vi "BuildPlotLegends_LSI218.vi"(8 "Plot selecter (2)\n    1      2     3     5":bool[][](array[boolean])=[[FALSE, TRUE, FALSE, FALSE], [FALSE, FALSE, FALSE, FALSE], [FALSE, FALSE, FALSE, FALSE], [FALSE, FALSE, FALSE, TRUE], [TRUE, FALSE, FALSE, FALSE], [FALSE, FALSE, FALSE, FALSE], [FALSE, FALSE, FALSE, FALSE], [FALSE, TRUE, FALSE, FALSE], [FALSE, TRUE, FALSE, FALSE], [FALSE, TRUE, FALSE, FALSE], [FALSE, TRUE, FALSE, FALSE], [FALSE, FALSE, FALSE, FALSE], [FALSE, FALSE, FALSE, FALSE], [FALSE, FALSE, FALSE, FALSE], [FALSE, FALSE, FALSE, FALSE], [FALSE, FALSE, FALSE, FALSE], [FALSE, FALSE, FALSE, FALSE], [FALSE, FALSE, FALSE, FALSE], [FALSE, FALSE, FALSE, FALSE], [FALSE, FALSE, FALSE, FALSE], [FALSE, FALSE, FALSE, FALSE], [FALSE, FALSE, FALSE, FALSE], [FALSE, FALSE, FALSE, FALSE], [FALSE, FALSE, FALSE, FALSE]], 9 "Plot selecter (1)\n    1      2     3     4":bool[][](array[boolean])=[[FALSE, TRUE, FALSE, FALSE], [FALSE, FALSE, FALSE, FALSE], [FALSE, FALSE, FALSE, FALSE], [FALSE, FALSE, FALSE, TRUE], [TRUE, FALSE, FALSE, FALSE], [FALSE, FALSE, FALSE, FALSE], [FALSE, FALSE, FALSE, FALSE], [FALSE, TRUE, FALSE, FALSE], [FALSE, TRUE, FALSE, FALSE], [FALSE, TRUE, FALSE, FALSE], [FALSE, TRUE, FALSE, FALSE], [FALSE, FALSE, FALSE, FALSE], [FALSE, FALSE, FALSE, FALSE], [FALSE, FALSE, FALSE, FALSE], [FALSE, FALSE, FALSE, FALSE], [FALSE, FALSE, FALSE, FALSE], [FALSE, FALSE, FALSE, FALSE], [FALSE, FALSE, FALSE, FALSE], [FALSE, FALSE, FALSE, FALSE], [FALSE, FALSE, FALSE, FALSE], [FALSE, FALSE, FALSE, FALSE], [FALSE, FALSE, FALSE, FALSE], [FALSE, FALSE, FALSE, FALSE], [FALSE, FALSE, FALSE, FALSE]], 10 "Labels (2)":string[](array[string])=["B1", "B2", "B3", "B4", "B5"], 11 "Labels (1)":string[](array[string])=["A1", "A2", "A3", "A4", "A5"]) -> (0 "Series 4":string[](array[string])=["A4"], 1 "Series 3":string[](array[string]), 2 "Series 2":string[](array[string])=["A1", "B3", "B4", "B5"], 3 "Series 1":string[](array[string])=["A5"])   [LabVIEW 2017]
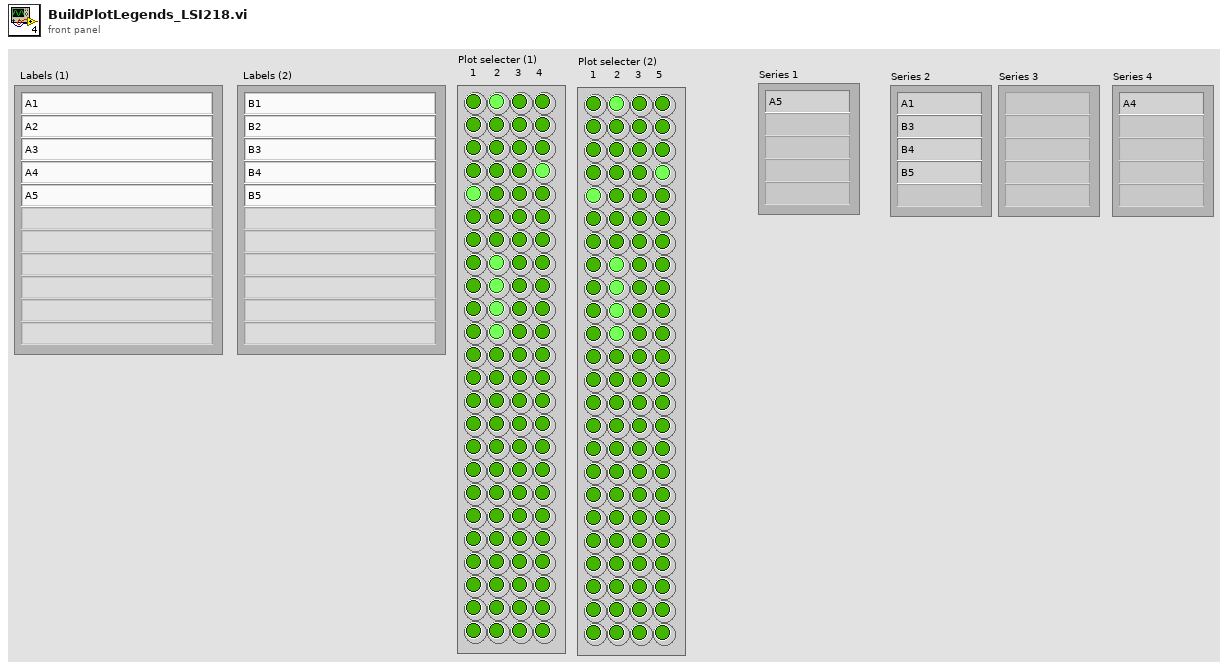
[diagram p1: front panel]
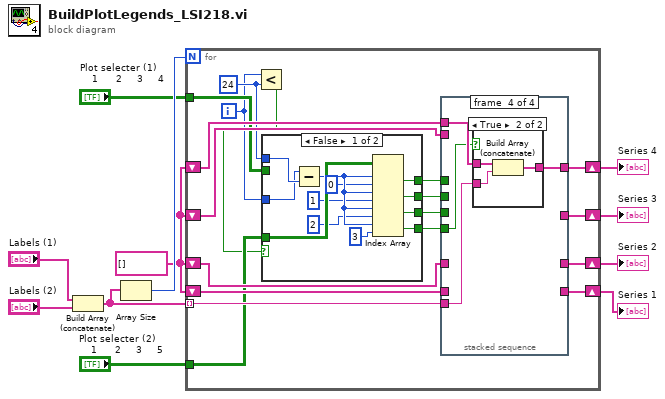
[diagram p0: block diagram]
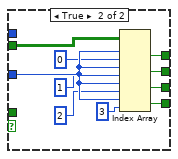
[diagram p2: hidden frame]
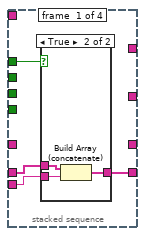
[diagram p3: hidden frame]
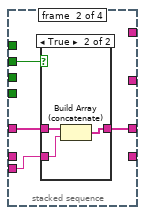
[diagram p5: hidden frame]
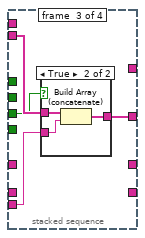
[diagram p7: hidden frame]
diagram:
  w9 = string[] []
  n1 = Build Array (concatenate)("Labels (1)", "Labels (2)") -> (w2:string[])
  n2 = Array Size(array=w2) -> (size(s)=w11:i32)
  n3 = for {
    N: w11 -> [_]
    shift-right: [w22] -> w8
    shift-left: w9 -> [w29]
    shift-right: [w24] -> w6
    shift-left: w9 -> [w28]
    shift-right: [w23] -> w7
    shift-left: w9 -> [w27]
    shift-right: [w21] -> w5
    shift-left: w9 -> [w26]
    tunnel: "Plot selecter (1)\n    1      2     3     4" -> [w19]
    tunnel: w2 -> [w25] mode=indexing
    tunnel: "Plot selecter (2)\n    1      2     3     5" -> [w18]
    i -> [w13]
    w20 = 24 ("y")
    n4 = Less?(x=w13, y=w20) -> (x < y?=w12:bool)
    n5 = case shown="False" w12 {
      tunnel: [w33 w51] -> w17
      tunnel: [w32 w50] -> w16
      tunnel: [w31 w48] -> w15
      tunnel: [w30 w47] -> w14
      tunnel: w20 -> [w40 _]
      tunnel: w19 -> [_ w46]
      tunnel: w18 -> [w39 _]
      tunnel: w13 -> [w34 w45]
      frame False {
        n6 = Subtract(x=w34, y=w40) -> (x-y=w38:i32)
        n7 = Index Array(array=w39, index (row) #1=w38, index (col) #1=0 ("index (row)"), index (row) #2=w38, index (col) #2=1 ("index (row)"), index (row) #3=w38, index (col) #3=2 ("index (row)"), index (row) #4=w38, index (col) #4=3 ("index (row)")) -> (element #1=w33:bool, element #2=w32:bool, element #3=w31:bool, element #4=w30:bool)
      }
      frame True {
        n8 = Index Array(array=w46, index (row) #1=w45, index (col) #1=0 ("index (row)"), index (row) #2=w45, index (col) #2=1 ("index (row)"), index (row) #3=w45, index (col) #3=2 ("index (row)"), index (row) #4=w45, index (col) #4=3 ("index (row)")) -> (element #1=w51:bool, element #2=w50:bool, element #3=w48:bool, element #4=w47:bool)
      }
    }
    n9 = stacked-sequence {
      tunnel: [w55 _ _ _] -> w22
      tunnel: [_ _ w71 _] -> w24
      tunnel: [_ _ _ w79] -> w21
      tunnel: w29 -> [w54 _ _ _]
      tunnel: w28 -> [_ _ w70 _]
      tunnel: [_ w63 _ _] -> w23
      tunnel: w27 -> [_ w62 _ _]
      tunnel: w26 -> [_ _ _ w78]
      tunnel: w25 -> [w53 w61 w69 w77]
      tunnel: w17 -> [w52 _ _ _]
      tunnel: w16 -> [_ w60 _ _]
      tunnel: w15 -> [_ _ w68 _]
      tunnel: w14 -> [_ _ _ w76]
      frame #0 {
        n10 = case shown="True" w52 {
          tunnel: [w56 w59] -> w55
          tunnel: w54 -> [w56 w58]
          tunnel: w53 -> [_ w57]
          frame False {
          }
          frame True {
            n11 = Build Array (concatenate)(w58, w57) -> (w59:string[])
          }
        }
      }
      frame #1 {
        n12 = case shown="True" w60 {
          tunnel: [w64 w67] -> w63
          tunnel: w62 -> [w64 w66]
          tunnel: w61 -> [_ w65]
          frame False {
          }
          frame True {
            n13 = Build Array (concatenate)(w66, w65) -> (w67:string[])
          }
        }
      }
      frame #2 {
        n14 = case shown="True" w68 {
          tunnel: [w72 w75] -> w71
          tunnel: w70 -> [w72 w74]
          tunnel: w69 -> [_ w73]
          frame False {
          }
          frame True {
            n15 = Build Array (concatenate)(w74, w73) -> (w75:string[])
          }
        }
      }
      frame #3 {
        n16 = case shown="True" w76 {
          tunnel: [w80 w83] -> w79
          tunnel: w78 -> [w80 w82]
          tunnel: w77 -> [_ w81]
          frame False {
          }
          frame True {
            n17 = Build Array (concatenate)(w82, w81) -> (w83:string[])
          }
        }
      }
    }
  }
  "Series 1" <- w8
  "Series 2" <- w7
  "Series 3" <- w6
  "Series 4" <- w5
